vi "SetValueNumeric.vi"(7 "LabVIEW Web Service Request":refnum<class "Web Request.lvclass">, 10 "ControlValue":dbl, 11 "ControlName":string="Start") -> (1 "Error":i32, 2 "ErrorString":string, 3 "dataOut":dbl)   [LabVIEW 2024]
uses:
  <vilib>/wsapi/Web Request.lvclass
  g_VIServerPort.vi
panel:
  out "value":string
  out "errorOut":errorcluster
  # "Use the Web Service Request input terminal to call the VIs on the Web Services palette. Do not remove it from the connector pane unless you don't need access to the palette."
  # "Each additional control wired to the connector pane will be available as an input in the URL. To include an indicator in terminal-mode output (the default setting), it must also be wired to the connector pane."
  # "http://127.0.0.1:8001/WebService/SetValueNumeric?ControlName={value}"
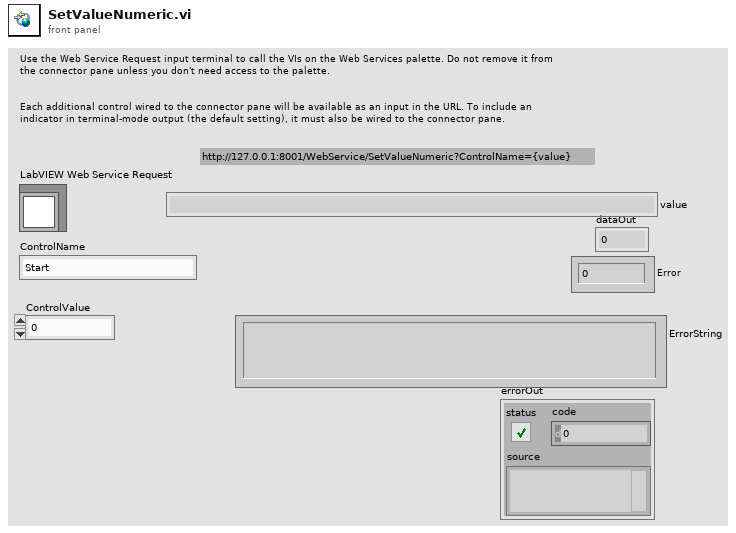
[diagram p1: front panel]
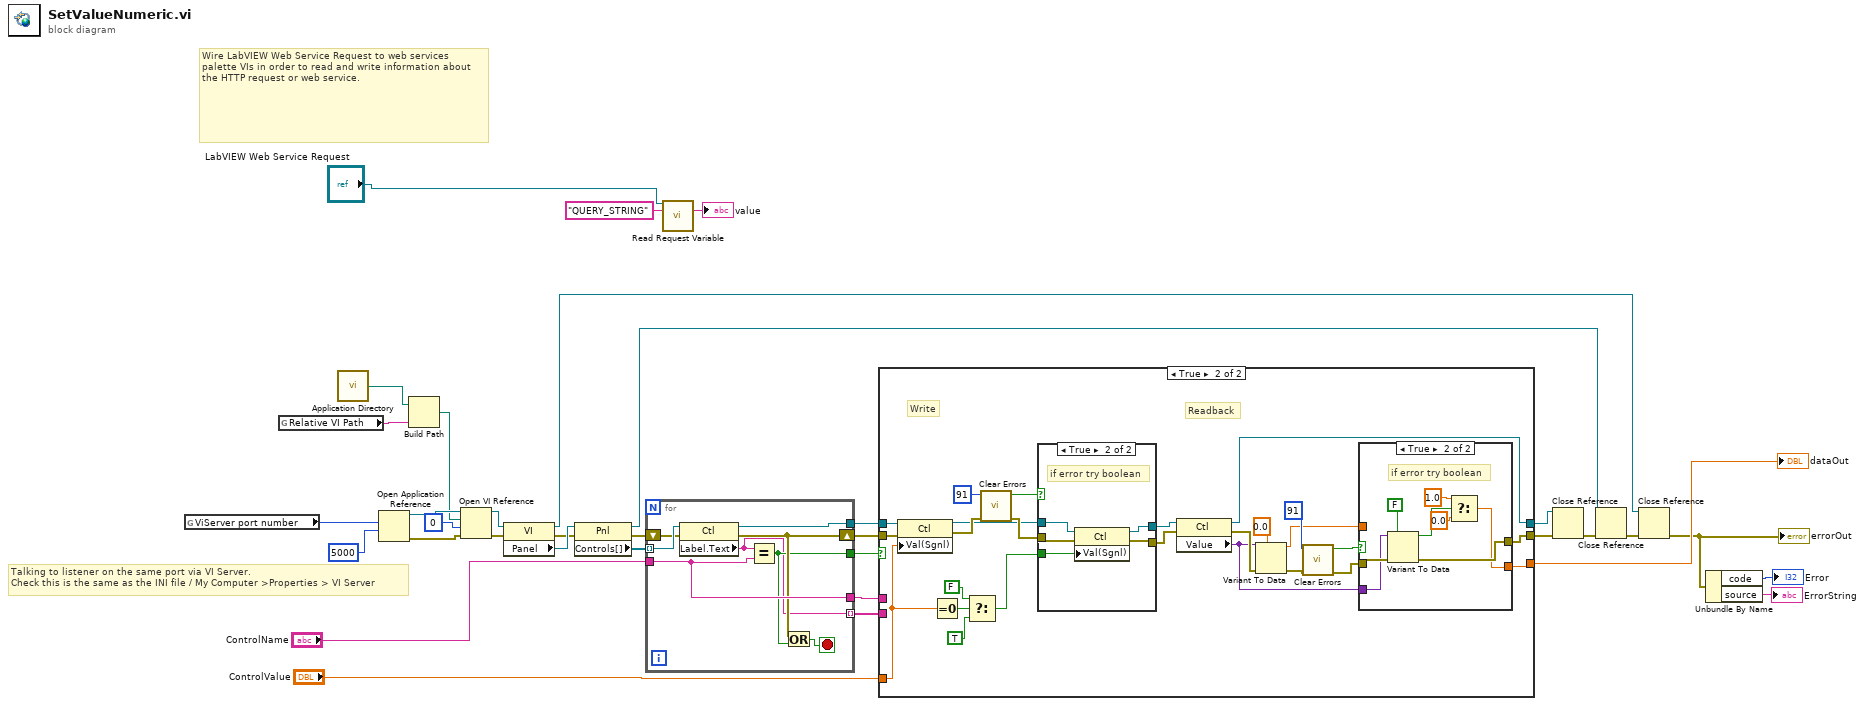
[diagram p0: block diagram]
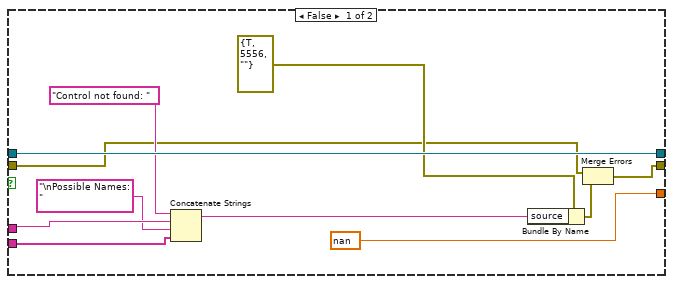
[diagram p2: hidden frame]
diagram:
  # "Talking to listener on the same port via VI Server.\nCheck this is the same as the INI file / My Computer >Properties > VI Server"
  # "Wire LabVIEW Web Service Request to web services palette VIs in order to read and write information about the HTTP request or web service."
  n1 = global read "g_VIServerPort.vi" "ViServer port number"() -> (w2:u16)
  n2 = global read "g_VIServerPort.vi" "Relative VI Path"() -> (w1:string)
  n3 = call <vilib>:"Application Directory.vi"() -> ("Application Directory"=w8:path)
  n4 = Open Application Reference(9:5000 ("timeout ms (60000)"), 10:w2) -> (0:w14:errorcluster, 3:w15:refnum<vi>)  [unwired: 2 in]
  n5 = Build Path(base path=w8, name or relative path=w1) -> (appended path=w7:path)
  n6 = Open VI Reference(application reference (local)=w15, vi path=w7, options=0, error in (no error)=w14) -> (vi reference=w18:refnum<vi>, error out=w30:errorcluster)  [unwired: 2 in]
  n7 = property class="VI"(reference=w18, error in=w30) -> (reference out=w25:refnum<vi>, error out=w29:errorcluster, "Panel"=w33:refnum<vi>)
  n8 = property class="Pnl"(reference=w33, error in=w29) -> (reference out=w19:refnum<vi>, error out=w28:errorcluster, "Controls[]"=w32:refnum<vi>[])
  n9 = for {
    tunnel: w32 -> [w42] mode=indexing
    tunnel: "ControlName" -> [w39]
    tunnel: [w36] -> w27
    tunnel: [w40] -> w20
    tunnel: [w39] -> w16
    shift-right: [w37] -> w21
    shift-left: w28 -> [w41]
    tunnel: [w35] -> w10 mode=indexing
    stop <- w38 stop-if-true
    n10 = property class="Ctl"(reference=w42, error in=w41) -> (reference out=w40:refnum<vi>, error out=w37:errorcluster, "Label.Text"=w35:string)
    n11 = Equal?(x=w35, y=w39) -> (x = y?=w36:bool)
    n12 = Or(x=w37, y=w36) -> (x .or. y?=w38:bool)
  }
  n13 = call <vilib>:"Read Request Variable.vi"("LabVIEW Web Service Request"="LabVIEW Web Service Request", "variable name"="QUERY_STRING") -> ("value"=→"value":string)  [unwired: 11 in, 2 out]
  n14 = case shown="True" w27 {
    tunnel: w20 -> [w53 w78]
    tunnel: [w53 w74] -> w26
    tunnel: [w47 w56] -> w22
    tunnel: w21 -> [w48 w77]
    tunnel: [nan ("Ctrl Val to set (Num)") w54] -> w17
    tunnel: w16 -> [w45 _]
    tunnel: w10 -> [w43 _]
    tunnel: "ControlValue" -> [_ w69]
    frame False {
      n15 = Concatenate Strings("Control not found: " ("string"), w45, "\nPossible Names: " ("string"), w43) -> (w51:string)
      n16 = Bundle By Name(cluster=errorcluster {"status"=TRUE, "code"=5556, "source"=""} ("error constant"), "source"=w51) -> (w49:errorcluster)
      n17 = Merge Errors(w48, w49) -> (w47:errorcluster)
    }
    frame True {
      # "Readback"
      # "Write"
      n18 = property class="Ctl"(reference=w78, error in=w77, "Val(Sgnl)"=w69) -> (reference out=w65:refnum<vi>, error out=w73:errorcluster)
      n19 = Equal To 0?(x=w69) -> (x = 0?=w68:bool)
      n20 = Select(t=FALSE, s=w68, f=TRUE) -> (s? t:f=w64:bool)
      n21 = call <vilib>:"Clear Errors.vi"("error in (no error)"=w73, "specific error code to clear (0: all)"=91) -> ("error out"=w70:errorcluster, "specific error cleared?"=w71:bool)  [unwired: 4 in]
      n22 = case shown="True" w71 {
        tunnel: [w90 w91] -> w62
        tunnel: w70 -> [w90 w95]
        tunnel: w65 -> [w89 w94]
        tunnel: w64 -> [_ w93]
        tunnel: [w89 w92] -> w63
        frame False {
        }
        frame True {
          # "if error try boolean"
          n23 = property class="Ctl"(reference=w94, error in=w95, "Val(Sgnl)"=w93) -> (reference out=w92:refnum<vi>, error out=w91:errorcluster)
        }
      }
      n24 = property class="Ctl"(reference=w63, error in=w62) -> (reference out=w74:refnum<vi>, error out=w75:errorcluster, "Value"=w57:variant)
      n25 = Variant To Data(error in=w75, type=0.0 ("Ctrl Val to set (Num)"), Variant=w57) -> (data=w55:dbl, error out=w61:errorcluster)
      n26 = call <vilib>:"Clear Errors.vi"("error in (no error)"=w61, "specific error code to clear (0: all)"=91) -> ("error out"=w60:errorcluster, "specific error cleared?"=w59:bool)  [unwired: 4 in]
      n27 = case shown="True" w59 {
        tunnel: [w80 w87] -> w56
        tunnel: w60 -> [w80 w88]
        tunnel: [w79 w84] -> w54
        tunnel: w57 -> [_ w81]
        tunnel: w55 -> [w79 _]
        frame False {
        }
        frame True {
          # "if error try boolean"
          n28 = Variant To Data(error in=w88, type=FALSE, Variant=w81) -> (data=w85:bool, error out=w87:errorcluster)
          n29 = Select(t=1.0, s=w85, f=0.0) -> (s? t:f=w84:dbl)
        }
      }
    }
  }
  "dataOut" <- w17
  n30 = Close Reference(reference=w26, error in (no error)=w22) -> (error out=w24:errorcluster)
  n31 = Close Reference(reference=w19, error in (no error)=w24) -> (error out=w23:errorcluster)
  n32 = Close Reference(reference=w25, error in (no error)=w23) -> (error out=w13:errorcluster)
  "errorOut" <- w13
  n33 = Unbundle By Name(w13) -> ("code"=→"Error":i32, "source"=→"ErrorString":string)
